vi "Config Scan Count.vi"(6 "Reset Coupled Parameters (true)":bool=TRUE, 7 "Mode (Each)":i32(ring) items=["Each", "Inner", "Second", "Third"], 8 "error in":errorcluster, 9 "Reset Count (true)":bool=TRUE, 10 "Total (0)":i32 min=0 max=99999999, 11 "VISA resource name":refnum<visa-resource-name>) -> (0 "error out":errorcluster, 3 "VISA resource name out":refnum<visa-resource-name>)   [LabVIEW 2017, in "Andeen-Hagerling 2700.lvlib"]
doc: "This VI configures the scan parameters. This includes Scan Total, Scan Mode, Reset Count and Reset Coupled Parameters."
uses:
  Andeen-Hagerling 2700.lvlib
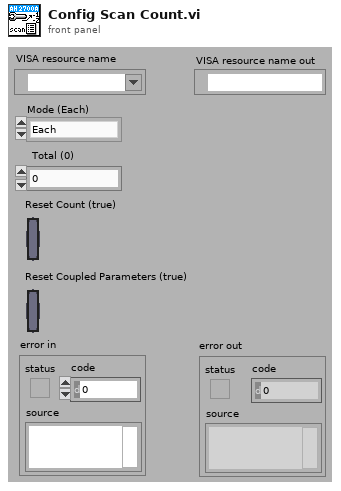
[diagram p1: front panel]
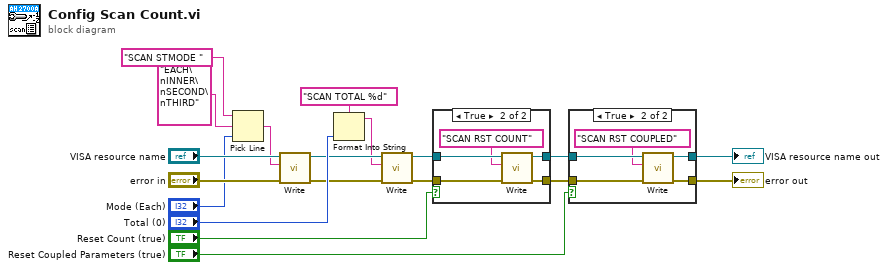
[diagram p0: block diagram]
diagram:
  n1 = Pick Line(string ("")="SCAN STMODE ", multi-line string="EACH\nINNER\nSECOND\nTHIRD", line index="Mode (Each)") -> (output string=w14:string)
  n2 = call "Write.vi"("error in"="error in", "command"=w14, "VISA resource name"="VISA resource name") -> ("error out"=w10:errorcluster, "VISA resource name out"=w11:refnum<visa-resource-name>)  [unwired: 7 in]
  n3 = Format Into String(format string="SCAN TOTAL %d", "Total (0)") -> (resulting string=w9:string)  [unwired: 2 in, 1 out]
  n4 = call "Write.vi"("error in"=w10, "command"=w9, "VISA resource name"=w11) -> ("error out"=w7:errorcluster, "VISA resource name out"=w8:refnum<visa-resource-name>)  [unwired: 7 in]
  n5 = case shown="True" "Reset Count (true)" {
    tunnel: w8 -> [w21 w26]
    tunnel: [w21 w25] -> w5
    tunnel: w7 -> [w20 w24]
    tunnel: [w20 w23] -> w3
    frame False {
    }
    frame True {
      n6 = call "Write.vi"("error in"=w24, "command"="SCAN RST COUNT", "VISA resource name"=w26) -> ("error out"=w23:errorcluster, "VISA resource name out"=w25:refnum<visa-resource-name>)  [unwired: 7 in]
    }
  }
  n7 = case shown="True" "Reset Coupled Parameters (true)" {
    tunnel: w5 -> [w28 w33]
    tunnel: [w28 w32] -> w4
    tunnel: w3 -> [w27 w31]
    tunnel: [w27 w30] -> w2
    frame False {
    }
    frame True {
      n8 = call "Write.vi"("error in"=w31, "command"="SCAN RST COUPLED", "VISA resource name"=w33) -> ("error out"=w30:errorcluster, "VISA resource name out"=w32:refnum<visa-resource-name>)  [unwired: 7 in]
    }
  }
  "VISA resource name out" <- w4
  "error out" <- w2
